vi "Robot Global Data.vi"() -> ()   [LabVIEW 2018]
doc: "This global VI can contain as many global variables as you need. Place a control on the panel, give it a good name. To read or write to it from a VI, drag the icon to the diagram of that VI. You can also drag from the project. Click on the node to change which global you access. You shouldn't have multiple locations writing to a global or it will cause a race-condition."
uses:
  <vilib>/Rock Robotics/WPI/Camera/WPI_CameraImageSize.ctl
  <vilib>/Rock Robotics/WPI/DriverStation/WPI_DriverStationRobotMode2.ctl
  <vilib>/Rock Robotics/WPI/ThirdParty/Phoenix-LabVIEW/CANifier/CTRE_CANifier_PWMChannel.ctl
panel:
  out "Max Motor Output":dbl=0.5
  in  "Panel Routine Running":bool
  in  "Cancel Panel Routine":bool
  in  "kMotorController":T1
  in  "Robot Mode":T2
  in  "image size":T3=enum."320x240"
  in  "Enable Vision":bool
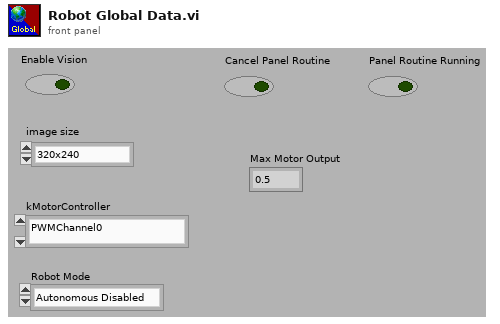
[diagram p1: front panel]
types:
  T1 = typedef "CTRE_CANifier_PWMChannel.ctl" = enum16{"PWMChannel0", "PWMChannel1", "PWMChannel2", "PWMChannel3"}
  T2 = typedef "WPI_DriverStationRobotMode2.ctl" = enum16{"Autonomous Disabled", "Autonomous Enabled", "Teleop Disabled", "Teleop Enabled", "Disconnected", "Finish", "Test Disabled", "Test Enabled", "Emergency Stopped"}
  T3 = typedef "WPI_CameraImageSize.ctl" = enum16{"640x480", "320x240", "160x120", "Custom"}
diagram:
